vi "Update.vi"(11 "Proto in":refnum<class "Heat Map.lvclass">) -> (3 "Proto out":refnum<class "Heat Map.lvclass">)   [LabVIEW 2021, in "Heat Map.lvclass"]
uses:
  Heat Map.lvclass
  Heat Map.lvclass/Heat Map.ctl
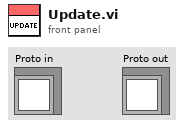
[diagram p1: front panel]
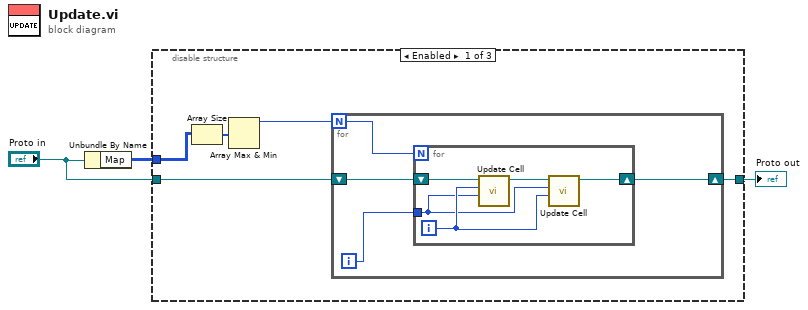
[diagram p0: block diagram]
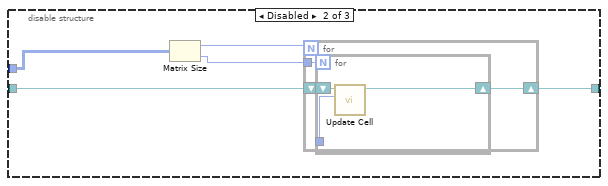
[diagram p2: hidden frame]
diagram:
  n1 = Unbundle By Name("Proto in") -> ("Map"=w3:i32[][])
  n2 = disable-structure shown="Enabled" {
    disable-tunnel: w3 -> [w8 w20 _]
    disable-tunnel: "Proto in" -> [w7 w22 _]
    disable-tunnel: [w6 w21 _] -> w1
    frame Enabled {
      n3 = Array Size(array=w8) -> (size(s)=w5:i32[])
      n4 = Array Max & Min(array=w5) -> (max value=w4:i32)  [unwired: 3 out]
      n5 = for {
        N: w4 -> [w9]
        shift-right: [w11] -> w6
        shift-left: w7 -> [w12]
        i -> [w10]
        n6 = for {
          N: w9 -> [_]
          shift-right: [w15] -> w11
          shift-left: w12 -> [w17]
          tunnel: w10 -> [w13]
          i -> [w14]
          n7 = call "Update Cell.vi"("Col"=w13, "Row"=w14, "Heat Map in"=w17) -> ("Heat Map out"=w16:refnum<class "Heat Map.lvclass">)  [unwired: 8 in]
          n8 = call "Update Cell.vi"("Col"=w14, "Row"=w13, "Heat Map in"=w16) -> ("Heat Map out"=w15:refnum<class "Heat Map.lvclass">)  [unwired: 8 in]
        }
      }
    }
    frame Disabled {
      n9 = Matrix Size(0:w20) -> (1:w19:i32, 2:w18:i32)
      n10 = for {
        N: w19 -> [_]
        shift-right: [w25] -> w21
        shift-left: w22 -> [w26]
        tunnel: w18 -> [w24]
        i -> [w23]
        n11 = for {
          N: w24 -> [_]
          shift-right: [w29] -> w25
          shift-left: w26 -> [w30]
          tunnel: w23 -> [w28]
          i -> [w27]
          n12 = call "Update Cell.vi"("Col"=w27, "Row"=w28, "Heat Map in"=w30) -> ("Heat Map out"=w29:refnum<class "Heat Map.lvclass">)  [unwired: 8 in]
        }
      }
    }
    frame Disabled {
    }
  }
  "Proto out" <- w1
